vi "5302GetSensitivityVISA.vi"(8 "error in (no error)":errorcluster, 11 "VISA session (for class)":refnum<visa-resource-name>) -> (0 "error out":errorcluster, 1 "data string":string, 2 "Sevsitivity":dbl format="%.4e", 3 "VISA session":refnum<visa-resource-name>)   [LabVIEW 2015]
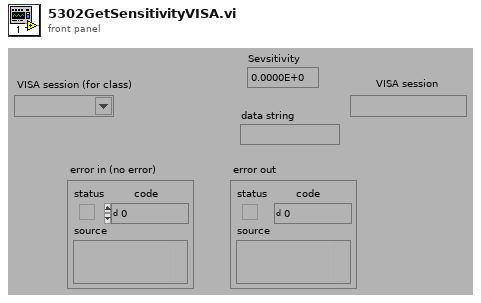
[diagram p1: front panel]
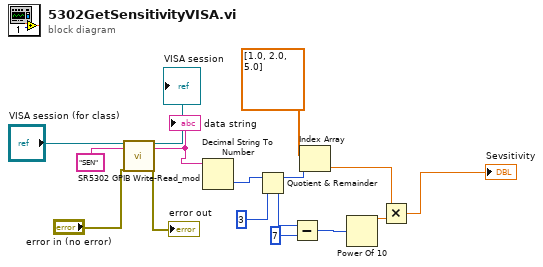
[diagram p0: block diagram]
diagram:
  n1 = call "SR5302 GPIB Write-Read_mod.vi"("VISA session (for class)"="VISA session (for class)", "Write Command String"="SEN" ("data string"), "error in (no error)"="error in (no error)") -> ("VISA session"=→"VISA session":refnum<visa-resource-name>, "Response 1"=w2:string, "error out"=→"error out":errorcluster)  [unwired: 5 in, 9 out]
  "data string" <- w2
  n2 = Decimal String To Number(string=w2) -> (number=w10:i32)  [unwired: 2 in, 1 out]
  n3 = Quotient & Remainder(x=w10, y=3) -> (x-y*floor(x/y)=w6:i32, floor(x/y)=w8:i32)
  n4 = Subtract(x=w8, y=7) -> (x-y=w9:i32)
  n5 = Index Array(array=dbl[] [1.0, 2.0, 5.0] ("Input Array"), index=w6) -> (element=w4:dbl)
  n6 = Power Of 10(x=w9) -> (10^x=w12:dbl)
  n7 = Multiply(x=w4, y=w12) -> (x*y=→"Sevsitivity":dbl)
